vi "qREC DAT.vi"(0 "System no.":i32=1 min=1 max=4 step=1, 1 "RecorderID":string, 2 "RecorderFormat":string="ASCII", 3 "StartPoint":i32 min=1 max=4 step=1, 4 "NumberOfPoints":i32 min=1 max=4 step=1, 5 "error in":errorcluster, 7 "TraceID":i32 min=1 max=4 step=1) -> (14 "Recorded data as GCSArray":string, 19 "error out":errorcluster)   [LabVIEW 2020]
doc: "REC? DAT (Get Recorded Data Values)\n\nDescription\nReads the recorded data points from the traces of a data recorder\n\nFormat\nREC? DAT <RecorderID> <RecorderFormat>[ <StartPoint>[ <NumberOfPoints>[{ <TraceID>}]]]\n\nArguments\n<RecorderID>\nData recorder to be queried; to be specified as alias (p. 94) \nThe available data recorders can be queried with USG? SYS (p. 80). \nPossible values: REC_1 to RECn, where n = number of data recorders in the controller\n<RecorderFormat>\nData format in which the data is to be transmitted \nThe supported data formats can be queried with USG? PROP (p. 79). \nPossible values: ASCII\n<StartPoint>\nIndex of the data point from which the data is to be read out\nThe number of data points recorded per trace of the data recorder can be queried with REC? \nNUM (p. 45). \nPossible values:\n>= 1\nMaximum value = Number of recorded points\n<NumberOfPoints>\nNumber of data points that is to be read out per trace\nPossible values:\n>= 1\nMaximum value = Number of recorded points -<StartPoint> + 1\n<TraceID>\nID of the trace to be read out\nThe number of traces of the data recorder can be queried via parameter 0x104. Example:\n>>spv? ram rec_1 - 0x104\n<<RAM REC_1 - 0x104=4\nThe trace to be read out must contain recorded data. Otherwise, the reading out with REC? DAT \nfails and the controller reports an error.\nFor a trace to be able to record data, it must have been configured beforehand, i.e. a parameter \nto be recorded must be assigned to it. In order to find out which traces can be read out, it is \ntherefore useful to first query with REC? TRACE (p. 48) to find out which traces are configured \nfor recording. \nNote that the data in all traces of a data recorder will be deleted if the configuration for a trace \nis changed. See the state diagram for the data recorder (p. 110). \nPossible values: 1 to n, where n = Number of traces of the data recorder\n\nResponse\nThe recorded data in GCS array format\nThe header for the output of the recorded data must have at least the following content:\n<<# IDN = (c)2018-2021 Physik Instrumente (PI) SE & Co. KG,\nUMF-DEMO, 0000000000, 0.13.3.0\n<<# REC_ID = <RecorderID>\n<<# VERSION = 1 \n<<# TYPE = 1 \n<<# SEPARATOR = 9 \n<<# DIM = <NumberOfTraces>\n<<# NDATA = <NumberOfPoints>\n<<# SAMPLE_TIME = <SampleTime>\n<<# TRIGGER_TIME = <TriggerStartTime>\n<<# \n{# NAME<N> = <ParameterDescription> (<CU> <FU> <ParameterId>)}\n<<# END_HEADER\n- <NumberOfTraces>: Number of read traces\n- <NumberOfPoints>: Number of read data points per trace\n- <SampleTime>: Product of the recording rate of the data recorder and the servo cycle \ntime of the controller\n- <TriggerStartTime>: System time of the trigger event in milliseconds\nIf at least one of the queried traces contains no data, the response will consist of a line feed \n(ASCII character 0x0A) and the controller will report an error.\nIf <TraceID> is left out, all of the traces on the data recorder that contain recorded data will be \nread. The scope of the response depends on the arguments used with the REC? DAT command:\n- If only <RecorderID> and <RecorderFormat> are specified, all of the recorded data \npoints will be output.\n- If <RecorderID>, <RecorderFormat> and <StartPoint> are specified, all of the recorded \ndata points from the stated start point onwards will be output.\n- If <RecorderID>, <RecorderFormat>, <StartPoint> and <NumberOfPoints> are specified, \nthe stated number of data points will be output from the stated start point onwards.\nIf <TraceID> is specified, the stated number of data points for this trace will be output from the \nstated start point onwards.\nIn the response, the queried traces will be sorted in data columns according to their TraceIDs in \nascending order.\n\nNotes\nFor further details, see \"Data Recorder - GCS 3.0\" (p. 107). \n\nUser command level\nUSR"
panel:
  # "REC? DAT (Get Recorded Data Values)\n\nReads the recorded data points from the traces of a data recorder."
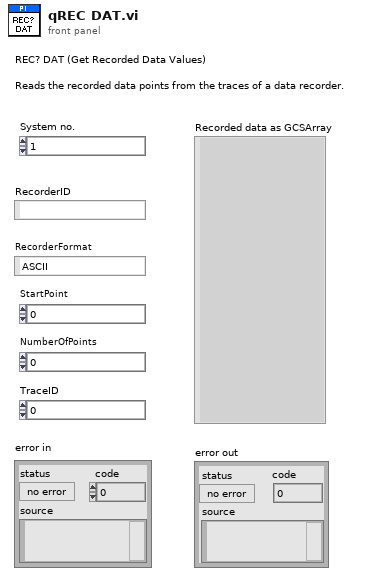
[diagram p1: front panel]
types:
  T1 = typedef "Syntax.ctl" = enum16{"GCS 1.0", "GCS 2.0", "GCS 3.0"}
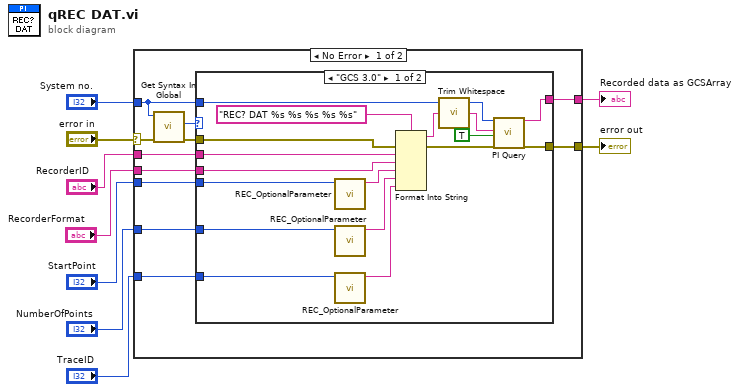
[diagram p0: block diagram]
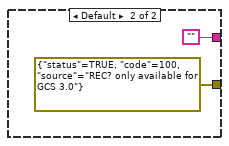
[diagram p2: hidden frame]
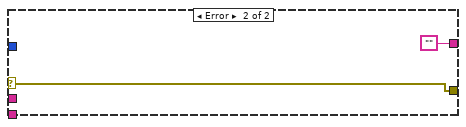
[diagram p3: hidden frame]
diagram:
  n1 = case shown="No Error" "error in" {
    selector: "error in" -> [w18 w41]
    tunnel: [w17 w41] -> w8
    tunnel: "NumberOfPoints" -> [w11 _]
    tunnel: "StartPoint" -> [w13 _]
    tunnel: "TraceID" -> [w12 _]
    tunnel: "System no." -> [w10 _]
    tunnel: [w15 ""] -> w3
    tunnel: "RecorderID" -> [w16 _]
    tunnel: "RecorderFormat" -> [w14 _]
    frame No Error {
      n2 = call "Get Syntax In Global.vi"("error in"=w18, "System no."=w10) -> ("error out"=w19:errorcluster, "Syntax"=w20:T1)  [unwired: 8 in]
      n3 = case shown="\"GCS 3.0\"" w20 {
        tunnel: [w31 errorcluster {"status"=TRUE, "code"=100, "source"="REC? only available for GCS 3.0"} ("error out")] -> w17
        tunnel: w19 -> [w36 _]
        tunnel: w16 -> [w35 _]
        tunnel: w14 -> [w34 _]
        tunnel: [w29 ""] -> w15
        tunnel: w13 -> [w28 _]
        tunnel: w12 -> [w21 _]
        tunnel: w11 -> [w23 _]
        tunnel: w10 -> [w26 _]
        frame "GCS 3.0" {
          n4 = call "REC_OptionalParameter.vi"("Number"=w28) -> ("String"=w27:string)  [unwired: 10 in]
          n5 = call "REC_OptionalParameter.vi"("Number"=w23) -> ("String"=w24:string)  [unwired: 10 in]
          n6 = call "REC_OptionalParameter.vi"("Number"=w21) -> ("String"=w22:string)  [unwired: 10 in]
          n7 = Format Into String(format string="REC? DAT %s %s %s %s %s", error in=w36, w35, w34, w27, w24, w22) -> (resulting string=w33:string, error out=w30:errorcluster)  [unwired: 1 in]
          n8 = call <vilib>:"Trim Whitespace.vi"("string"=w33) -> ("trimmed string"=w25:string)  [unwired: 1 in]
          n9 = call "PI Query.vi"("System no."=w26, "String to send"=w25, "Attach termination char.?"=TRUE ("Attach Linefeed?"), "error in"=w30) -> ("String read"=w29:string, "error out"=w31:errorcluster)  [unwired: 3 in, 11 out]
        }
        frame Default {
        }
      }
    }
    frame Error {
    }
  }
  "error out" <- w8
  "Recorded data as GCSArray" <- w3
